vi "add_light-dark_jt_to_queue.vi"(10 "Scan settings array":T3[](array[typedef]) {"Settling delay (s)" min=0.0; "J-t illumination" items=["Light only", "Dark only", "Light then dark", "Dark then light"]; "Measurement speed" items=["Fast", "Normal", "High accuracy"]; "Illumination" items=["Light only", "Dark only", "Light then dark", "Dark then light"]; "Only repeat for best pixel" items=["only for best pixel", "for best 2 pixels", "for best 3 pixels", "for best 4 pixels", "for best 5 pixels", "for best 6 pixels", "for best 7 pixels", "for all pixels"]; "No. of repeat scans" min=1.0 step=1.0; "Max power best pixel only" items=["only the best pixel", "the best 2 pixels", "the best 3 pixels", "the best 4 pixels", "the best 5 pixels", "the best 6 pixels", "the best 7 pixels", "all pixels"]; "J-t best pixel only" items=["only the best pixel", "the best 2 pixels", "the best 3 pixels", "the best 4 pixels", "the best 5 pixels", "the best 6 pixels", "the best 7 pixels", "all pixels"]; "J-t measurement speed" items=["Fast", "Normal", "High Accuracy"]; "Stabilisation mode" items=["V", "I"]; "Measurement delay (s)" min=0.01}, 11 "Cell settings cluster":T2) -> (3 "Light/dark array":T1(array[cluster]))   [LabVIEW 2016]
uses:
  TypeDefs/scan_settings.ctl
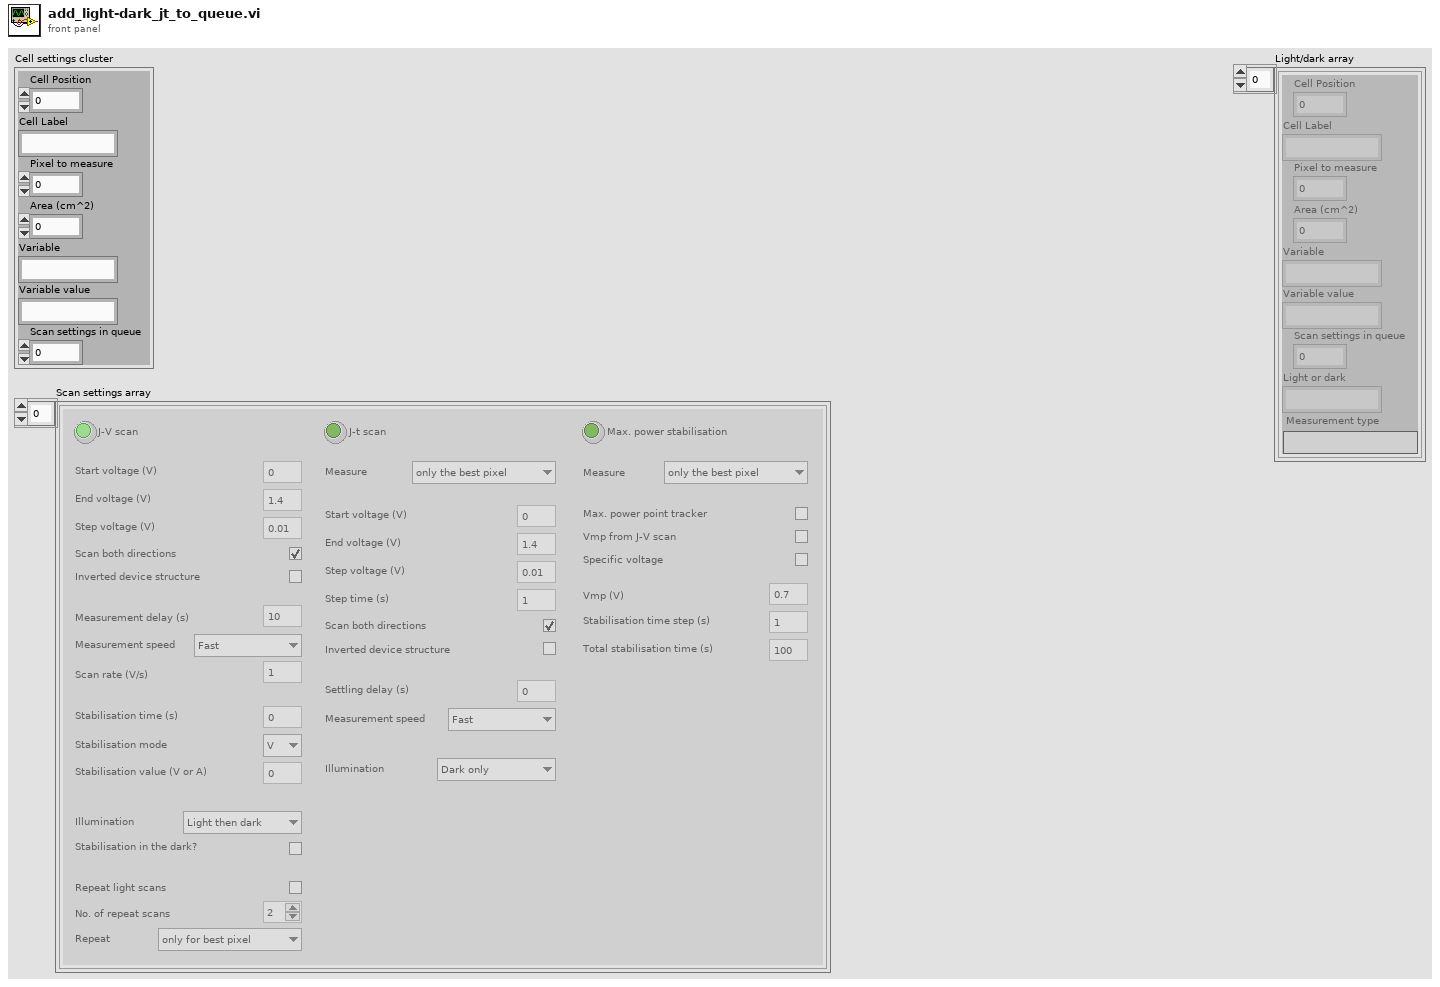
[diagram p1: front panel]
types:
  T1 = cluster{"Cell Position":i32, "Cell Label":string, "Pixel to measure":u16, "Area (cm^2)":dbl, "Variable":string, "Variable value":string, "Scan settings in queue":u16, "Light or dark":string, "Measurement type":string}[]
  T2 = cluster{"Cell Position":i32, "Cell Label":string, "Pixel to measure":u16, "Area (cm^2)":dbl, "Variable":string, "Variable value":string, "Scan settings in queue":u16}
  T3 = typedef "scan_settings.ctl" = cluster{"J-V scan":bool, "Start voltage (V)":dbl, "End voltage (V)":dbl, "Step voltage (V)":dbl, "Scan both directions":bool, "Inverted device structure":bool, "Measurement delay (s)":dbl, "Measurement speed":u8, "Scan rate (V/s)":dbl, "Stabilisation time (s)":dbl, "Stabilisation mode":u16, "Stabilisation value (V or A) ":dbl, "Illumination":u16, "Stabilisation in the dark?":bool, "Repeat light scans":bool, "No. of repeat scans":dbl, "Only repeat for best pixel":u16, "J-t scan":bool, "J-t best pixel only":u16, "J-t start voltage (V)":dbl, "J-t end voltage (V)":dbl, "J-t step voltage (V)":dbl, "Step time (s)":dbl, "J-t scan both directions":bool, "J-t inverted device structure":bool, "Settling delay (s)":dbl, "J-t measurement speed":u16, "J-t illumination":u16, "Max. power stabilisation":bool, "Max power best pixel only":u16, "Max. power point tracker":bool, "Vmp from J-V scan":bool, "Max P stab. Specific voltage":bool, "Vmp (V)":dbl, "Stabilisation time step (s)":dbl, "Total stabilisation time (s)":dbl}
  T4 = cluster{"Cell Position":i32, "Cell Label":string, "Pixel to measure":u16, "Area (cm^2)":dbl, "Variable":string, "Variable value":string, "Scan settings in queue":u16, "Light or dark":string, "Measurement type":string}
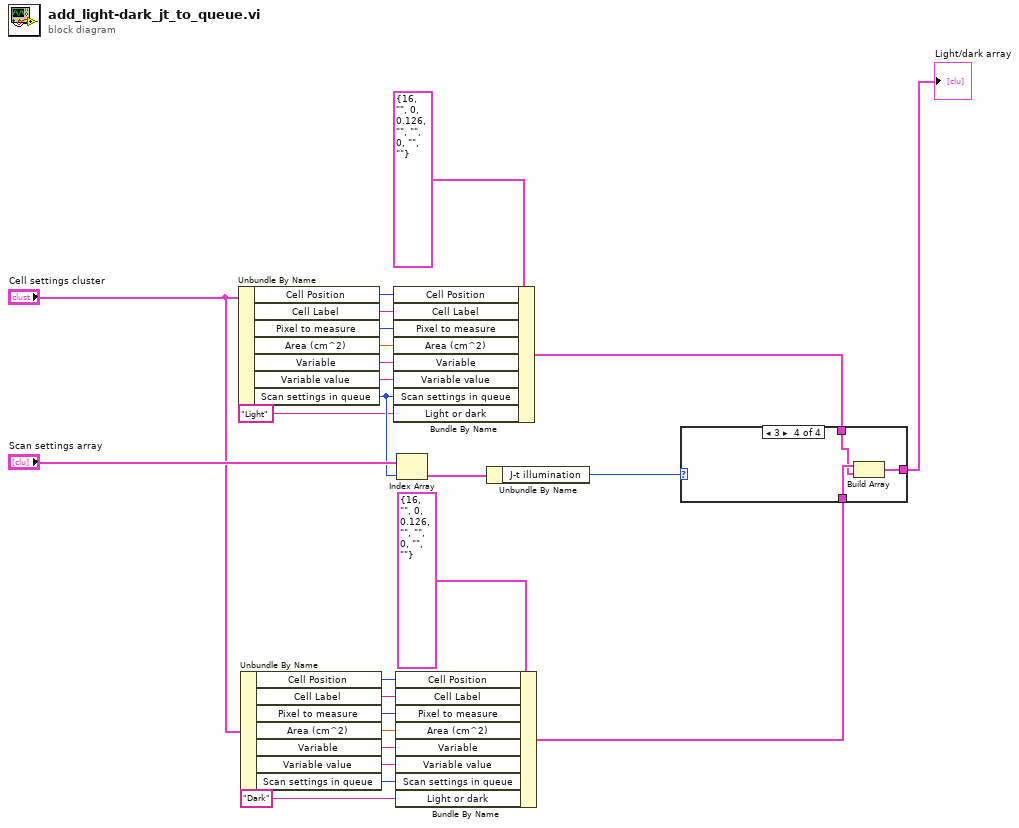
[diagram p0: block diagram]
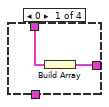
[diagram p2: hidden frame]
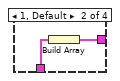
[diagram p3: hidden frame]
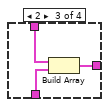
[diagram p4: hidden frame]
diagram:
  n1 = Unbundle By Name("Cell settings cluster") -> ("Cell Position"=w5:i32, "Cell Label"=w6:string, "Pixel to measure"=w7:u16, "Area (cm^2)"=w8:dbl, "Variable"=w9:string, "Variable value"=w10:string, "Scan settings in queue"=w23:u16)
  n2 = Unbundle By Name("Cell settings cluster") -> ("Cell Position"=w12:i32, "Cell Label"=w13:string, "Pixel to measure"=w14:u16, "Area (cm^2)"=w15:dbl, "Variable"=w16:string, "Variable value"=w17:string, "Scan settings in queue"=w18:u16)
  n3 = Bundle By Name(cluster=T4 {"Cell Position"=16, "Cell Label"="", "Pixel to measure"=0, "Area (cm^2)"=0.126, "Variable"="", "Variable value"="", "Scan settings in queue"=0, "Light or dark"="", "Measurement type"=""} ("System Cluster"), "Cell Position"=w5, "Cell Label"=w6, "Pixel to measure"=w7, "Area (cm^2)"=w8, "Variable"=w9, "Variable value"=w10, "Scan settings in queue"=w23, "Light or dark"="Light") -> (w3:T4)
  n4 = Bundle By Name(cluster=T4 {"Cell Position"=16, "Cell Label"="", "Pixel to measure"=0, "Area (cm^2)"=0.126, "Variable"="", "Variable value"="", "Scan settings in queue"=0, "Light or dark"="", "Measurement type"=""} ("System Cluster"), "Cell Position"=w12, "Cell Label"=w13, "Pixel to measure"=w14, "Area (cm^2)"=w15, "Variable"=w16, "Variable value"=w17, "Scan settings in queue"=w18, "Light or dark"="Dark") -> (w20:T4)
  n5 = Index Array(array="Scan settings array", index=w23) -> (element=w25:T3)
  n6 = Unbundle By Name(w25) -> ("J-t illumination"=w1:u16)
  n7 = case shown="3" w1 {
    tunnel: w3 -> [w27 _ w32 w33]
    tunnel: w20 -> [_ w29 w30 w35]
    tunnel: [w26 w28 w31 w34] -> w21
    frame 0 {
      n8 = Build Array(w27) -> (w26:T1)
    }
    frame 1, Default {
      n9 = Build Array(w29) -> (w28:T1)
    }
    frame 2 {
      n10 = Build Array(w32, w30) -> (w31:T1)
    }
    frame 3 {
      n11 = Build Array(w35, w33) -> (w34:T1)
    }
  }
  "Light/dark array" <- w21
